vi "ReverseCurrentRead.vi"(6 "Reset":bool, 10 "Switch Direction":bool) -> (2 "Reverse Read":bool)   [LabVIEW 2014]
panel:
  # "Copyright 2014 Vidrio Technologies\nScanImage 5 software is licensed under the Apache License, Version 2.0 (the \"License\"); you may not use any files contained\nwithin the ScanImage 5 release except in compliance with the License. You may obtain a copy of the License at\n http://www.apache.org/licenses/LICENSE-2.0\nUnless required by applicable law or agreed to in writing, software distributed under the License is distributed on an\n\"AS IS\" BASIS, WITHOUT WARRANTIES OR CONDITIONS OF ANY KIND, either express or implied. See the License for the\n specific language governing permissions and limitations under the License."
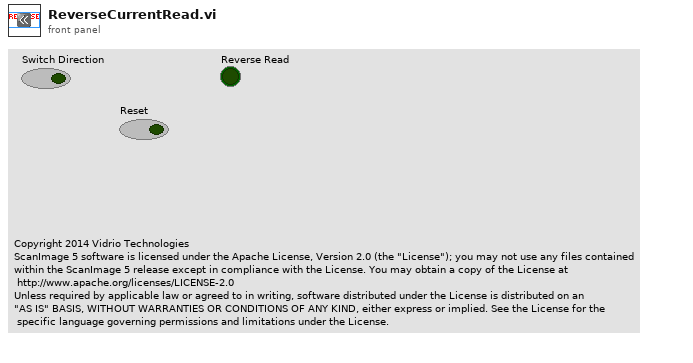
[diagram p1: front panel]
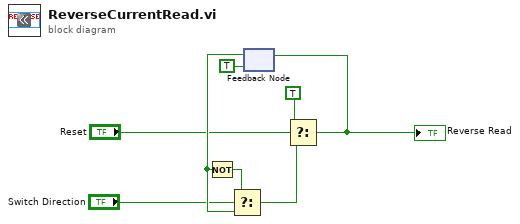
[diagram p0: block diagram]
diagram:
  n1 = feedback #1(TRUE) -> (w7:bool)
  n2 = Not(x=w7) -> (.not. x?=w8:bool)
  n3 = Select(t=w8, s="Switch Direction", f=w7) -> (s? t:f=w1:bool)
  n4 = Select(t=TRUE, s="Reset", f=w1) -> (s? t:f=w5:bool)
  "Reverse Read" <- w5
  n5 = feedback-in #1(w5) -> ()
